vi "Test 4 Get Symbol Position.vi"(8 "error in (no error)":errorcluster, 11 "Test Case In":refnum<class "Schema parsing test.lvclass">) -> (0 "error out":errorcluster, 3 "Test Case Out":refnum<class "Schema parsing test.lvclass">)   [LabVIEW 2020, in "Schema parsing test.lvclass"]
uses:
  Schema parsing test.lvclass
  4993e8ee-a06a-463a-9684-69129f64d5ce.vi
  Symbol/Symbol.lvclass
  9da8f5d6-6cef-4195-a5ac-e87968932722.vi
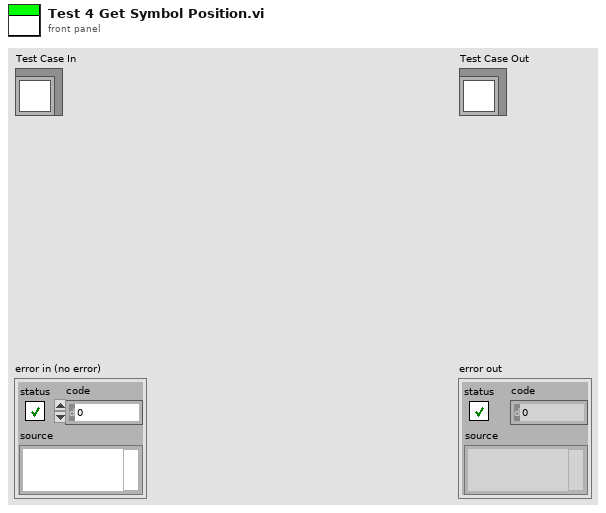
[diagram p1: front panel]
types:
  T1 = typedef "Symbol.lvclass/Coordinate.ctl" = cluster{"Col":i32, "Row":i32}
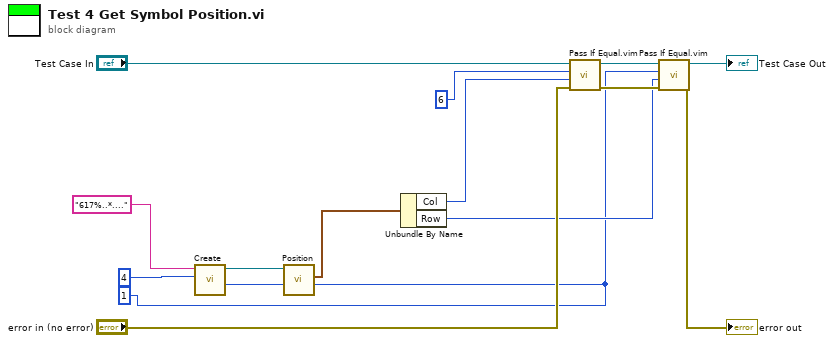
[diagram p0: block diagram]
diagram:
  w1 = 1 ("Row")
  n1 = call "Create.vi"("Row"=w1, "Col Offset"=4, "String"="617%..*....") -> ("Number"=w9:refnum<class "Symbol.lvclass">)  [unwired: 6 in, 2 out]
  n2 = call "Position.vi"("Number in"=w9) -> ("Position"=w8:T1)  [unwired: 8 in, 2 out]
  n3 = Unbundle By Name(w8) -> ("Col"=w6:i32, "Row"=w2:i32)
  n4 = call "Pass If Equal.vim"("error in (no error)"="error in (no error)", "Actual"=w6, "Expected"=6 ("Col"), "LUnit Test Case In"="Test Case In") -> ("error out"=w12:errorcluster, "LUnit Test Case Out"=w4:refnum<class "Schema parsing test.lvclass">)  [unwired: 6 in]
  n5 = call "Pass If Equal.vim"("error in (no error)"=w12, "Actual"=w2, "Expected"=w1, "LUnit Test Case In"=w4) -> ("error out"=→"error out":errorcluster, "LUnit Test Case Out"=→"Test Case Out":refnum<class "Schema parsing test.lvclass">)  [unwired: 6 in]
